vi "AFT Get FIR Filtered-X Coefficients.vi"(8 "error in (no error)":errorcluster, 11 "filtered-x adaptive filter in":refnum<k20>) -> (0 "error out":errorcluster, 2 "coefficients":dbl[](array[numeric]), 3 "filtered-x adaptive filter out":refnum<k20>)   [LabVIEW 2017, in "NI_AdaptiveFilter.lvlib"]
doc: "Retrieves the coefficients from an adaptive filter that you create with the AFT Create FIR Filtered-X LMS or AFT Create FIR Normalized Filtered-X LMS VI."
uses:
  <vilib>/addons/Adaptive Filters/NI_AdaptiveFilter.lvlib
  <resource>/AdaptiveFilters.dll
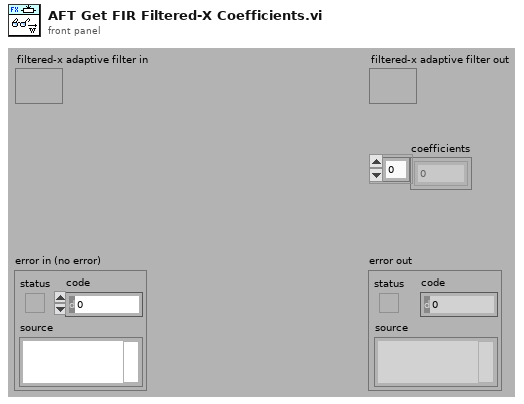
[diagram p1: front panel]
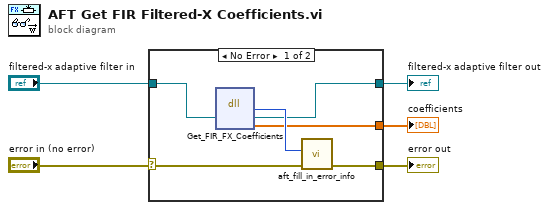
[diagram p0: block diagram]
diagram:
  n1 = case shown="No Error" "error in (no error)" {
    selector: "error in (no error)" -> [w11 w13]
    tunnel: [w9 w13] -> w5
    tunnel: "filtered-x adaptive filter in" -> [w7 w12]
    tunnel: [w6 w12] -> w2
    tunnel: [w8 _] -> w1
    frame No Error {
      n2 = dll-call lib="C:/Program Files/National Instruments/LabVIEW 2017/resource/AdaptiveFilters.dll" fn="Get_FIR_FX_Coefficients"("pSession"=w7) -> ("err"=w10:i32, "pSession"=w6:refnum<k20>, "Coefficients"=w8:dbl[])  [unwired: 3 in, 3 out]
      n3 = call <vilib>:"aft_fill_in_error_info.vi"("error in"=w11, "status code"=w10) -> ("error out"=w9:errorcluster)  [unwired: 2 in, 7 out]
    }
    frame Error {
    }
  }
  "error out" <- w5
  "filtered-x adaptive filter out" <- w2
  "coefficients" <- w1
